vi "PlotCantParams.vi"() -> ()   [LabVIEW 2014]
uses:
  TypeDefs/RectHatch.ctl
  TypeDefs/PowerSpeed.ctl
  <vilib>/Utility/file.llb/Read From Spreadsheet File (DBL).vi
panel:
  out "OH":T1(array[cluster])=[{-30.0, 30.0, 382.0, 300.0, 114.6, 229.2, 229.2, 382.0, 382.0}, {-15.0, 30.0, 382.0, 300.0, 95.5, 191.0, 286.5, 382.0, 382.0}, {0.0, 30.0, 327.0, 150.0, 98.1, 196.2, 196.2, 327.0, 327.0}, {15.0, 30.0, 382.0, 300.0, 114.6, 229.2, 229.2, 382.0, 382.0}, {30.0, 30.0, 382.0, 300.0, 152.8, 191.0, 229.2, 267.4, 382.0}, {-30.0, 15.0, 382.0, 300.0, 95.5, 191.0, 286.5, 382.0, 382.0}, {-15.0, 15.0, 327.0, 150.0, 81.75, 163.5, 245.25, 327.0, 327.0}, {0.0, 15.0, 382.0, 300.0, 152.8, 191.0, 229.2, 267.4, 382.0}, {15.0, 15.0, 327.0, 150.0, 130.8, 163.5, 196.2, 228.9, 327.0}, {30.0, 15.0, 382.0, 300.0, 114.6, 229.2, 229.2, 382.0, 382.0}, {-30.0, 0.0, 327.0, 150.0, 98.1, 196.2, 196.2, 327.0, 327.0}, {-15.0, 0.0, 382.0, 300.0, 95.5, 191.0, 286.5, 382.0, 382.0}, {0.0, 0.0, 327.0, 150.0, 81.75, 163.5, 245.25, 327.0, 327.0}, {15.0, 0.0, 382.0, 300.0, 152.8, 191.0, 229.2, 267.4, 382.0}, {30.0, 0.0, 327.0, 150.0, 130.8, 163.5, 196.2, 228.9, 327.0}, {-30.0, -15.0, 382.0, 300.0, 114.6, 229.2, 229.2, 382.0, 382.0}, {-15.0, -15.0, 327.0, 150.0, 98.1, 196.2, 196.2, 327.0, 327.0}, {0.0, -15.0, 382.0, 300.0, 95.5, 191.0, 286.5, 382.0, 382.0}, {15.0, -15.0, 327.0, 150.0, 81.75, 163.5, 245.25, 327.0, 327.0}, {30.0, -15.0, 382.0, 300.0, 152.8, 191.0, 229.2, 267.4, 382.0}, {-30.0, -30.0, 382.0, 300.0, 114.6, 229.2, 229.2, 382.0, 382.0}, {-15.0, -30.0, 382.0, 300.0, 95.5, 191.0, 286.5, 382.0, 382.0}, {0.0, -30.0, 327.0, 150.0, 130.8, 163.5, 196.2, 228.9, 327.0}, {15.0, -30.0, 382.0, 300.0, 152.8, 191.0, 229.2, 267.4, 382.0}, {30.0, -30.0, 327.0, 150.0, 98.1, 196.2, 196.2, 327.0, 327.0}]
  in  "DummyCubeLoc":cluster{dbl, dbl}={-45.0, 30.0}
  in  "Save?":bool
  in  "Path":path=path "\\\\nif-prgms-srvr.llnl.gov\\LMOT/Damage Group/Matthews/AM/fraunhofer SLM/BuildFiles_STL_ILT/SCN/OHparam_11-18-16"
  in  "HighPower":dbl=500.0
  in  "Display":T2={"Mode"=enum."Inherit Value", "PointSize"=1.0, "LineWidth"=1.0}
  in  "LayerEnd":u32=170
  in  "LayerStart":u32=170
  in  "HatchPow":T3={"Power"=300.0, "Mark Speed"=400.0, "Jump Speed"=1000.0}
  in  "RectHatch":T4={"Width"=10.0, "Height"=10.0, "Angle"=45.0, "OffX"=0.1, "OffY"=0.1, "Spacing"=0.1} {"Spacing" format="%#_13g"; "OffY" format="%#_13g"; "OffX" format="%#_13g"; "Height" format="%#_13g"; "Width" format="%#_13g"}
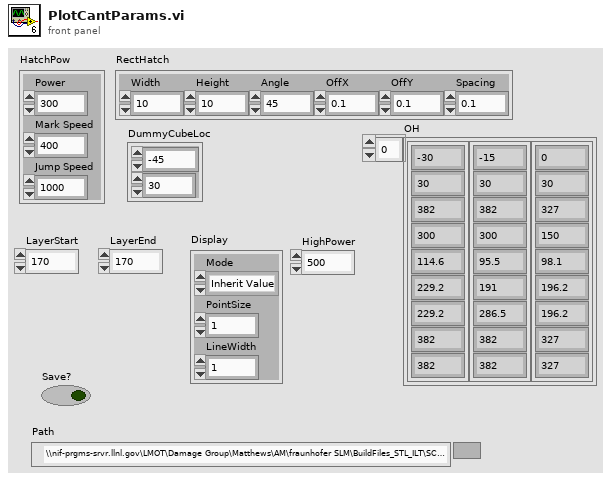
[diagram p1: front panel]
types:
  T1 = cluster{dbl, dbl, dbl, dbl, dbl, dbl, dbl, dbl, dbl}[]
  T2 = cluster{"Mode":enum16{"Inherit Value", "Points", "Wireframe", "Polygons"}, "PointSize":sgl, "LineWidth":sgl}
  T3 = typedef "PowerSpeed.ctl" = cluster{"Power":dbl, "Mark Speed":dbl, "Jump Speed":dbl}
  T4 = typedef "RectHatch.ctl" = cluster{"Width":dbl, "Height":dbl, "Angle":sgl, "OffX":dbl, "OffY":dbl, "Spacing":dbl}
  T5 = cluster{dbl, dbl, dbl, dbl, dbl, dbl, dbl, dbl, dbl}
  T6 = typedef "PathSupreme.ctl" = cluster{"VelocityProfiles":T7[], "Path":T8}
  T7 = typedef "VelocityProfile.ctl" = cluster{"ID":u32, "Velocity":dbl, "Mode":string, "tV1":u32, "tV2":u32, "tL1":u32, "tL2":u32}
  T8 = typedef "PathCut.ctl" = cluster{"Type":string, "Tag":string, "Segments":T9[]}
  T9 = typedef "Segment.ctl" = cluster{"SegmentID":u16, "Power":sgl, "idxVelocityProfile":u16, "End":cluster{"X":sgl, "Y":sgl}}
  T10 = typedef "Point3D.ctl" = cluster{"X":sgl, "Y":sgl, "Z":sgl}
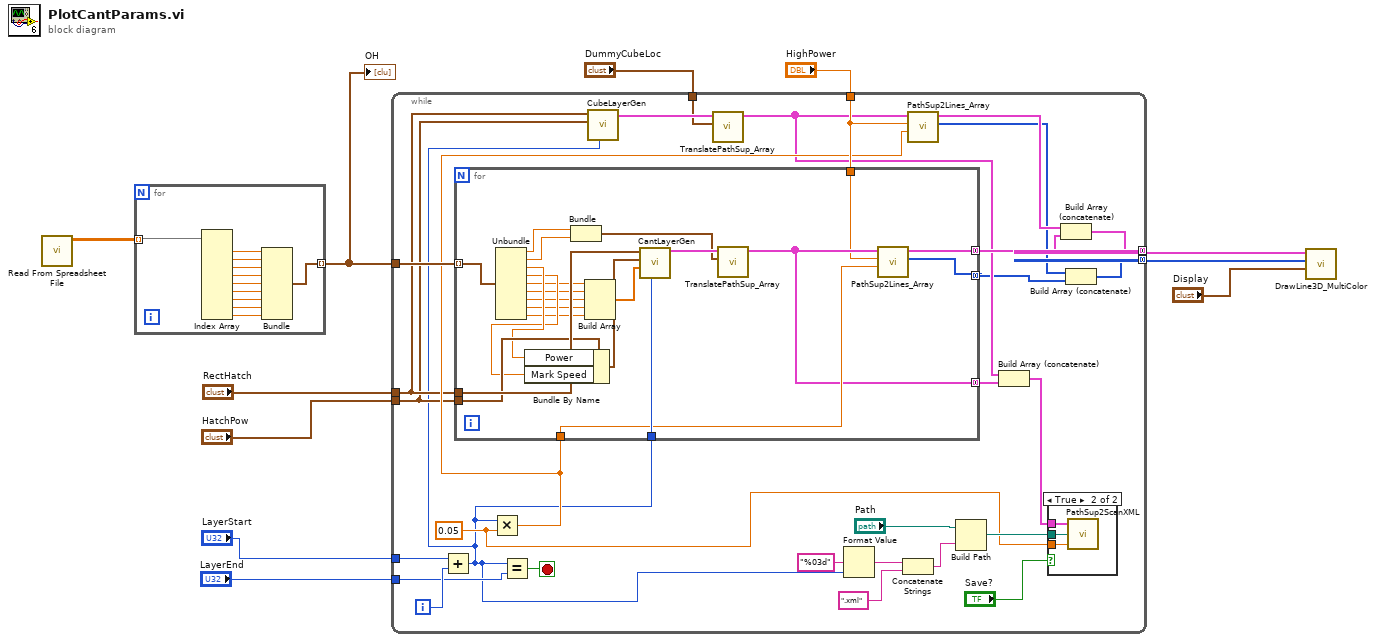
[diagram p0: block diagram]
diagram:
  n1 = call-poly <vilib>:"Read From Spreadsheet File.vi"() -> ("all rows"=w11:dbl[][])  [unwired: 7 in, 4 out]
  n2 = for {
    tunnel: w11 -> [w22] mode=indexing
    tunnel: [w17] -> w6 mode=indexing
    n3 = Index Array(array=w22) -> (element #1=w20:dbl, element #2=w21:dbl, element #3=w19:dbl, element #4=w18:dbl, element #5=w16:dbl, element #6=w15:dbl, element #7=w14:dbl, element #8=w13:dbl, element #9=w12:dbl)  [unwired: 9 in]
    n4 = Bundle(w20, w21, w19, w18, w16, w15, w14, w13, w12) -> (w17:T5)  [unwired: 1 in]
  }
  "OH" <- w6
  n5 = while {
    tunnel: "HighPower" -> [w36]
    tunnel: [w32] -> w9 mode=concatenating
    tunnel: [w31] -> w8 mode=concatenating
    tunnel: w6 -> [w49]
    tunnel: "RectHatch" -> [w27]
    tunnel: "HatchPow" -> [w26]
    tunnel: "LayerEnd" -> [w48]
    tunnel: "LayerStart" -> [w47]
    tunnel: "DummyCubeLoc" -> [w37]
    i -> [w51]
    stop <- w50 stop-if-true
    w40 = 0.05 ("y")
    n6 = Add(x=w47, y=w51) -> (x+y=w25:u32)
    n7 = Multiply(x=w25, y=w40) -> (x*y=w35:dbl)
    n8 = for {
      tunnel: w25 -> [w76]
      tunnel: w35 -> [w70]
      tunnel: w36 -> [w66]
      tunnel: [w75] -> w33 mode=concatenating
      tunnel: w49 -> [w74] mode=indexing
      tunnel: w27 -> [w73]
      tunnel: w26 -> [w64]
      tunnel: [w67] -> w30 mode=concatenating
      tunnel: [w65] -> w24 mode=concatenating
      n9 = Unbundle(w74) -> (w72:dbl, w71:dbl, w62:dbl, w61:dbl, w60:dbl, w59:dbl, w58:dbl, w57:dbl, w56:dbl)
      n10 = Bundle By Name(cluster=w64, "Power"=w62, "Mark Speed"=w61) -> (w63:T3)
      n11 = Bundle(w72, w71) -> (w68:cluster{dbl, dbl})  [unwired: 1 in]
      n12 = Build Array(w60, w59, w58, w57, w56) -> (w55:dbl[])
      n13 = call "CantLayerGen.vi"("Layer"=w76, "OHpows"=w55, "HatchPow"=w63, "RectHatch"=w73) -> ("PathSups"=w69:T6[])  [unwired: 5 in, 2 out]
      n14 = call "TranslatePathSup_Array.vi"("Offset"=w68, "PathSupsIn"=w69) -> ("PathSupsOut"=w67:T6[])  [unwired: 9 in]
      n15 = call "PathSup2Lines_Array.vi"("Z"=w70, "HighPower"=w66, "PathSupIn"=w67) -> ("Colors"=w65:u32[], "Lines"=w75:cluster{"P0":T10, "P1":T10}[])  [unwired: 7 in]
    }
    n16 = Equal?(x=w25, y=w48) -> (x = y?=w50:bool)
    n17 = call "CubeLayerGen.vi"("Layer"=w25, "HatchPow"=w26, "RectHatch"=w27) -> ("PathSups"=w38:T6[])  [unwired: 8 in]
    n18 = call "TranslatePathSup_Array.vi"("Offset"=w37, "PathSupsIn"=w38) -> ("PathSupsOut"=w29:T6[])  [unwired: 9 in]
    n19 = Format Value(format string="%03d", value (0)=w25) -> (output string=w45:string)  [unwired: 1 in]
    n20 = Concatenate Strings(w45, ".xml" ("string")) -> (w43:string)
    n21 = call "PathSup2Lines_Array.vi"("Z"=w35, "HighPower"=w36, "PathSupIn"=w29) -> ("Colors"=w23:u32[], "Lines"=w34:cluster{"P0":T10, "P1":T10}[])  [unwired: 7 in]
    n22 = Build Path(base path="Path", name or relative path=w43) -> (appended path=w41:path)
    n23 = Build Array (concatenate)(w29, w30) -> (w28:T6[])
    n24 = case shown="True" "Save?" {
      tunnel: w28 -> [_ w54]
      tunnel: w41 -> [_ w53]
      tunnel: w40 -> [_ w52]
      frame False {
      }
      frame True {
        n25 = call "PathSup2ScanXML.vi"("Thickness"=w52, "Path"=w53, "PathSupremes"=w54) -> ()  [unwired: 2 in, 1 out]
      }
    }
    n26 = Build Array (concatenate)(w34, w33) -> (w32:cluster{"P0":T10, "P1":T10}[])
    n27 = Build Array (concatenate)(w23, w24) -> (w31:u32[])
  }
  n28 = call "DrawLine3D_MultiColor.vi"("Display"="Display", "Colors"=w8, "Lines"=w9) -> ()  [unwired: 9 in]
